vi "AutonDAD.vi"(9 "BAD UP":bool, 11 "BAD Output":T1) -> ()   [LabVIEW 2012]
uses:
  <vilib>/Rock Robotics/WPI/Relay/WPI_RelayValue.ctl
  Robot Global Data.vi
  <vilib>/Rock Robotics/WPI/Solenoid/Deprecated/WPI_SolenoidSetBool.vi
panel:
  out "BAD Output":T1
  # "For debugging, later use constant"
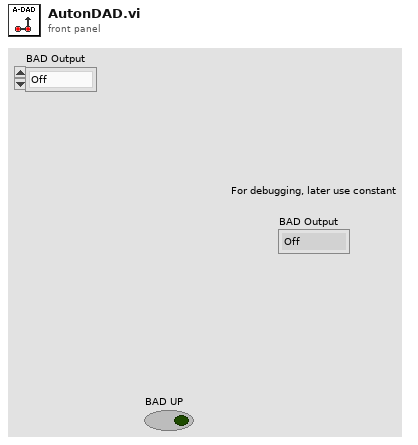
[diagram p1: front panel]
types:
  T1 = typedef "WPI_RelayValue.ctl" = enum16{"Off", "On", "Forward", "Reverse"}
  T2 = typedef "WPI_SolenoidDevRef.ctl" = cluster{"DevStatus":errorcluster, "Solenoid Module":T3, "Forward Solenoid Channel":T4, "Reverse Solenoid Channel":T4}
  T3 = typedef "FPGA_TypedefSolenoidModule.ctl" = enum16{"Solenoid Module 1", "Solenoid Module 2"}
  T4 = typedef "WPI_SolenoidChannel.ctl" = enum8{"Solenoid 1", "Solenoid 2", "Solenoid 3", "Solenoid 4", "Solenoid 5", "Solenoid 6", "Solenoid 7", "Solenoid 8", "Invalid"}
  T5 = typedef "WPI_RelayDevRef.ctl" = cluster{"DevStatus":errorcluster, "Relay Channel":T6, "Digital Module":T7, "Relay Direction":T8}
  T6 = typedef "FPGA_DIORelayChannel.ctl" = enum8{"Relay 1", "Relay 2", "Relay 3", "Relay 4", "Relay 5", "Relay 6", "Relay 7", "Relay 8", "Invalid"}
  T7 = typedef "FPGA_TypedefDigitalModule.ctl" = enum16{"Digital Module 1", "Digital Module 2"}
  T8 = typedef "WPI_RelayDirection.ctl" = enum16{"Both directions", "Forward only", "Reverse only"}
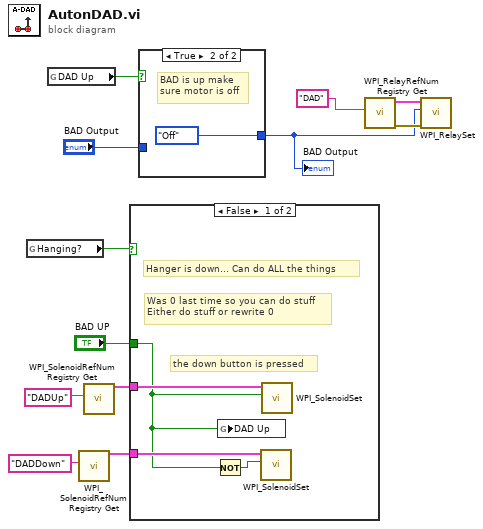
[diagram p0: block diagram]
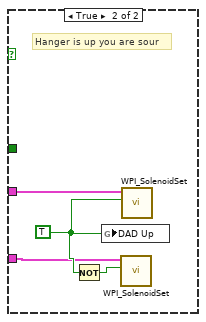
[diagram p2: hidden frame]
diagram:
  n1 = global read "Robot Global Data.vi" "Hanging?"() -> (w2:bool)
  n2 = global read "Robot Global Data.vi" "DAD Up"() -> (w9:bool)
  n3 = call <vilib>:"WPI_SolenoidRefNum Registry Get.vi"("refnum name"="DADDown") -> ("SolenoidDevRef"=w10:T2)  [unwired: 9 in, 1 out]
  n4 = call <vilib>:"WPI_SolenoidRefNum Registry Get.vi"("refnum name"="DADUp") -> ("SolenoidDevRef"=w11:T2)  [unwired: 9 in, 1 out]
  n5 = case shown="False" w2 {
    tunnel: w11 -> [w16 w18]
    tunnel: w10 -> [w15 w17]
    tunnel: "BAD UP" -> [w13 _]
    frame False {
      # "the down button is pressed"
      # "Was 0 last time so you can do stuff\nEither do stuff or rewrite 0"
      # "Hanger is down... Can do ALL the things"
      n6 = Not(x=w13) -> (.not. x?=w14:bool)
      n7 = global write "Robot Global Data.vi" "DAD Up"(w13) -> ()
      n8 = call-poly <vilib>:"WPI_SolenoidSet.vi"("Value"=w14, "SolenoidDevRef"=w15) -> ()  [unwired: 8 in, 2 out]
      n9 = call-poly <vilib>:"WPI_SolenoidSet.vi"("Value"=w13, "SolenoidDevRef"=w16) -> ()  [unwired: 8 in, 2 out]
    }
    frame True {
      w19 = TRUE
      # "Hanger is up you are sour"
      n10 = Not(x=w19) -> (.not. x?=w20:bool)
      n11 = global write "Robot Global Data.vi" "DAD Up"(w19) -> ()
      n12 = call-poly <vilib>:"WPI_SolenoidSet.vi"("Value"=w20, "SolenoidDevRef"=w17) -> ()  [unwired: 8 in, 2 out]
      n13 = call-poly <vilib>:"WPI_SolenoidSet.vi"("Value"=w19, "SolenoidDevRef"=w18) -> ()  [unwired: 8 in, 2 out]
    }
  }
  n14 = case shown="True" w9 {
    tunnel: [w21 WPI_RelayValue."Off" ("BAD Output")] -> w6
    tunnel: "BAD Output" -> [w21 _]
    frame False {
    }
    frame True {
      # "BAD is up make \nsure motor is off"
    }
  }
  "BAD Output" <- w6
  n15 = call <vilib>:"WPI_RelayRefNum Registry Get.vi"("refnum name"="DAD") -> ("error out"=w8:errorcluster, "RelayDevRef"=w7:T5)  [unwired: 9 in]
  n16 = call <vilib>:"WPI_RelaySet.vi"("error in (no error)"=w8, "RelayValue"=w6, "RelayDevRef"=w7) -> ()  [unwired: 7 in, 2 out]
